vi "SwapInstanceVIUnusedName2 53.vi"(6 "Bindata & descr in":T1, 7 "type":u16, 8 "error in (no error)":errorcluster, 9 "dims":u8=3 min=1 max=3, 11 "kwarg_name":string="testarg") -> (0 "error out":errorcluster, 1 "Array 3D":u16[][][](array[numeric]), 2 "Array 2D":u16[][](array[numeric]), 3 "Array 1D":u16[](array[numeric]), 4 "Bindata & descr out":T1, 5 "bindata":u8[](array[numeric]))   [LabVIEW 2018]
uses:
  Bindata&description.ctl
  Bindata description.ctl
  0361f700-1a3d-4472-b948-986616ee42e1.vi
  d71dc629-e1d7-4547-ad49-51f60279b8f3.vi
  0daf76d9-dc06-4993-b650-f6a506b52e1b.vi
  1b7006e8-8065-478a-ab9f-dd396f45bd52.vi
  d71dc629-e1d7-4547-ad49-51f60279b8f3.vi/124a42c7-fdaa-4985-96c6-2826b8061ed7.vi
  0daf76d9-dc06-4993-b650-f6a506b52e1b.vi/79bf908d-8900-4553-87bd-774a4cf3f70f.vi
  1b7006e8-8065-478a-ab9f-dd396f45bd52.vi/35eaf143-508a-445d-ad42-3601d79cf506.vi
  d71dc629-e1d7-4547-ad49-51f60279b8f3.vi/124a42c7-fdaa-4985-96c6-2826b8061ed7.vi/10b0e929-388e-432a-81e9-6b3ccf7048da.vi
  0daf76d9-dc06-4993-b650-f6a506b52e1b.vi/79bf908d-8900-4553-87bd-774a4cf3f70f.vi/b5175cd1-dfe1-466d-bc44-7e4a79158b1f.vi
  1b7006e8-8065-478a-ab9f-dd396f45bd52.vi/35eaf143-508a-445d-ad42-3601d79cf506.vi/b2337b23-40aa-456f-8446-f1de3277d4f4.vi
  d71dc629-e1d7-4547-ad49-51f60279b8f3.vi/124a42c7-fdaa-4985-96c6-2826b8061ed7.vi/10b0e929-388e-432a-81e9-6b3ccf7048da.vi/7c0e6055-a5c1-4a88-a702-5c542a8ccbc7.vi
  0daf76d9-dc06-4993-b650-f6a506b52e1b.vi/79bf908d-8900-4553-87bd-774a4cf3f70f.vi/b5175cd1-dfe1-466d-bc44-7e4a79158b1f.vi/71719c7a-77f9-4552-95c7-c7a4f08beba1.vi
  1b7006e8-8065-478a-ab9f-dd396f45bd52.vi/35eaf143-508a-445d-ad42-3601d79cf506.vi/b2337b23-40aa-456f-8446-f1de3277d4f4.vi/2debb03f-447f-4330-8ef9-6d44531691ec.vi
  check ID validity.vi
  LV-Julia_ZMQ-Roundtrip_lib.lvlib
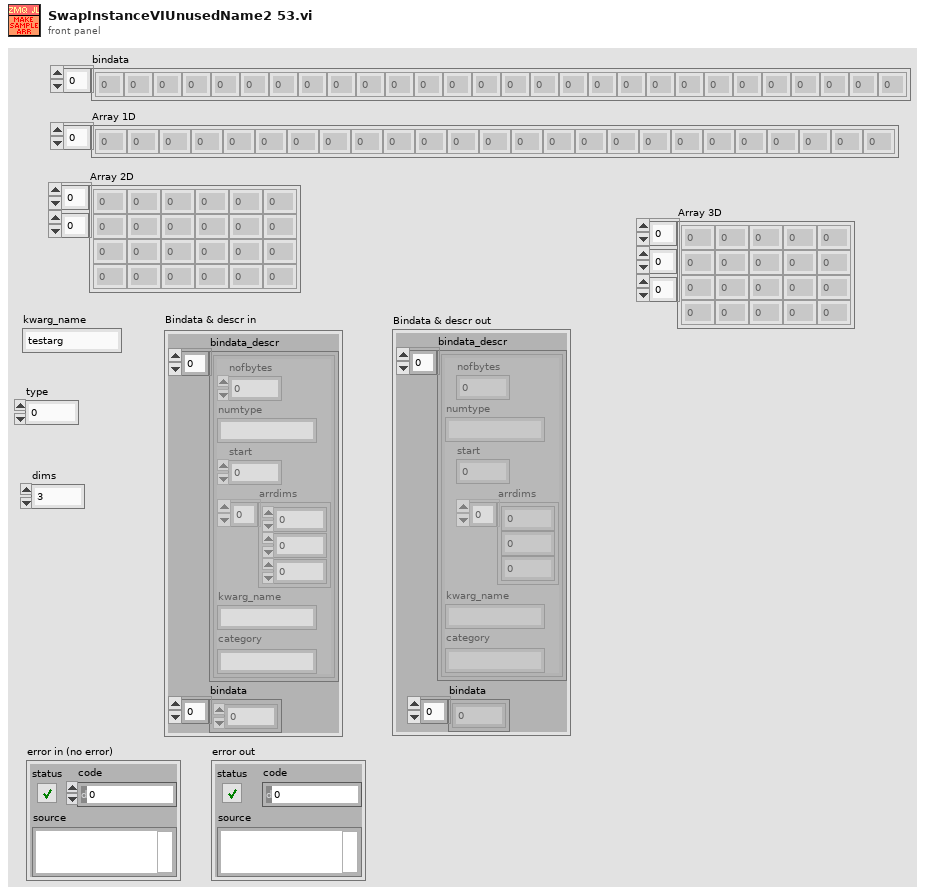
[diagram p1: front panel]
types:
  T1 = typedef "Bindata&description.ctl" = cluster{"bindata_descr":T2[], "bindata":u8[]}
  T2 = typedef "LV-Julia_ZMQ-Roundtrip_lib.lvlib/Bindata description.ctl" = cluster{"nofbytes":i32, "numtype":string, "start":i32, "arrdims":i32[], "kwarg_name":string, "category":string}
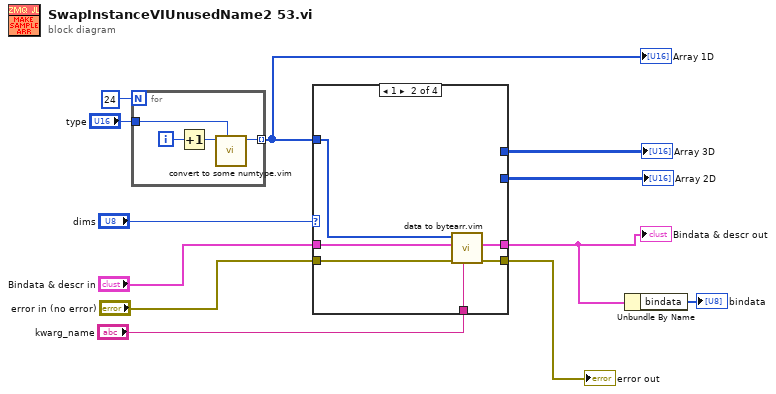
[diagram p0: block diagram]
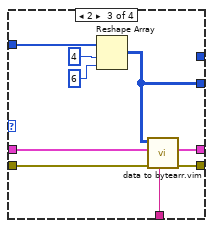
[diagram p3: hidden frame]
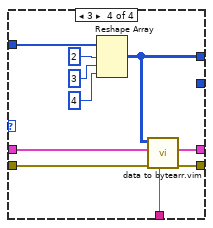
[diagram p4: hidden frame]
diagram:
  n1 = for {
    N: 24 -> [_]
    tunnel: [w14] -> w11 mode=indexing
    tunnel: "type" -> [w13]
    i -> [w16]
    n2 = Increment(x=w16) -> (x+1=w15:i32)
    n3 = call "convert to some numtype.vim"("type"=w13, "Numeric in"=w15) -> ("Numeric out"=w14:u16)  [unwired: 9 in]
  }
  "Array 1D" <- w11
  n4 = case shown="1" "dims" {
    tunnel: [_ _ _ w42] -> w12
    tunnel: w11 -> [_ w23 w30 w38]
    tunnel: "kwarg_name" -> [_ w22 w29 w37]
    tunnel: "error in (no error)" -> [w17 w21 w28 w36]
    tunnel: [w17 w20 w27 w35] -> w5
    tunnel: [_ w19 w26 w34] -> w2
    tunnel: [_ _ w25 _] -> w4
    tunnel: "Bindata & descr in" -> [_ w18 w24 w33]
    frame 0, Default {
    }
    frame 1 {
      n5 = call "data to bytearr.vim"("kwarg_name"=w22, "error in (no error)"=w21, "Bindata & descr in"=w18, "data in"=w23) -> ("error out"=w20:errorcluster, "Bindata & descr out"=w19:T1)  [unwired: 5 in, 1 out]
    }
    frame 2 {
      n6 = Reshape Array(w30, 4 ("dimension size"), 6 ("dimension size")) -> (w25:u16[][])
      n7 = call "data to bytearr.vim"("kwarg_name"=w29, "error in (no error)"=w28, "Bindata & descr in"=w24, "data in"=w25) -> ("error out"=w27:errorcluster, "Bindata & descr out"=w26:T1)  [unwired: 5 in, 1 out]
    }
    frame 3 {
      n8 = Reshape Array(w38, 2 ("dimension size"), 3 ("dimension size"), 4 ("dimension size")) -> (w42:u16[][][])
      n9 = call "data to bytearr.vim"("kwarg_name"=w37, "error in (no error)"=w36, "Bindata & descr in"=w33, "data in"=w42) -> ("error out"=w35:errorcluster, "Bindata & descr out"=w34:T1)  [unwired: 5 in, 1 out]
    }
  }
  "Array 3D" <- w12
  "Bindata & descr out" <- w2
  "error out" <- w5
  "Array 2D" <- w4
  n10 = Unbundle By Name(w2) -> ("bindata"=→"bindata":u8[])
